vi "Get w4lvgrpc_Msg_ToClient_3.vi"(8 "error in (no error)":errorcluster, 11 "gRPCid":T1) -> (0 "error out":errorcluster, 2 "package_templatemessage":T2, 3 "gRPCid out":T1)   [LabVIEW 2019, in "Generated_server.lvlib"]
uses:
  Generated_server.lvlib
  2ed25e12-861d-4677-8ead-ace2906b2041.vi
  w4lvgrpc_State.ctl
  w4lvgrpc_Msg_ToClient_3.ctl
  w4lvgrpc_Msg_ToClient_3_Flat.ctl
  <vilib>/gRPC/LabVIEW gRPC Library/Shared/grpcId.ctl
  <vilib>/gRPC/LabVIEW gRPC Library/grpc-lvsupport-release.lvlib
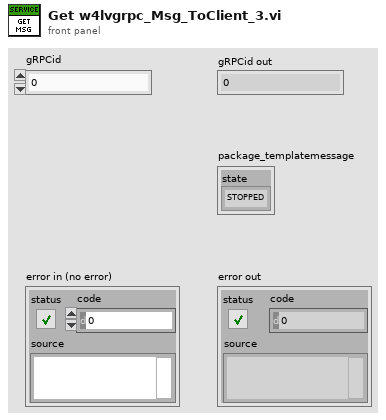
[diagram p1: front panel]
types:
  T1 = typedef "grpc-lvsupport-release.lvlib/grpcId.ctl" = u64
  T2 = typedef "Generated_server.lvlib/w4lvgrpc_Msg_ToClient_3.ctl" = cluster{"state":T3}
  T3 = typedef "Generated_server.lvlib/w4lvgrpc_State.ctl" = enum32{"STOPPED", "RUNNING", "ERROR"}
  T4 = typedef "Generated_server.lvlib/w4lvgrpc_Msg_ToClient_3_Flat.ctl" = cluster{"state":T3}
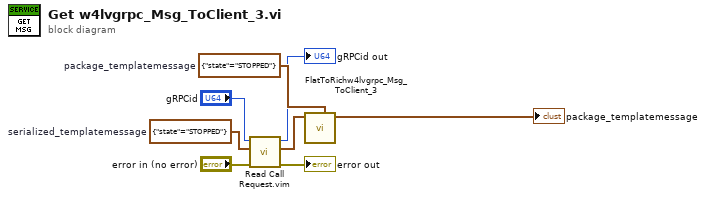
[diagram p0: block diagram]
diagram:
  w6 = T4 {"state"=enum."STOPPED"}  # serialized_templatemessage
  w5 = T2 {"state"=enum."STOPPED"}  # package_templatemessage
  n1 = call "Read Call Request.vim"("error in"="error in (no error)", "Request Type"=w6, "gRPCid in"="gRPCid") -> ("error out"=→"error out":errorcluster, "Request Data"=w4:T4, "gRPCid out"=→"gRPCid out":T1)  [unwired: 6 in]
  n2 = call "FlatToRichw4lvgrpc_Msg_ToClient_3.vi"("OutputClusterType"=w5, "InputCluster"=w4) -> ("OutputCluster"=→"package_templatemessage":T2)  [unwired: 9 in]
